vi "Read Last Known State.vi"(8 "error in (no error)":errorcluster, 11 "FP-TC-Shared.lvclass":refnum<class "FP-TC-Shared.lvclass">) -> (0 "error out":errorcluster, 1 "Last State Known":bool, 2 "LC Type":T1, 3 "FP-TC-Shared.lvclass":refnum<class "FP-TC-Shared.lvclass">)   [LabVIEW 2019, in "FP-TC-Shared.lvclass"]
uses:
  FP-TC-Shared.lvclass
  typedefs/LC Type--Enum.ctl
  FP-TC-Shared.lvclass/FP-TC-Shared.ctl
  <vilib>/Utility/config.llb/NI_LVConfig.lvlib
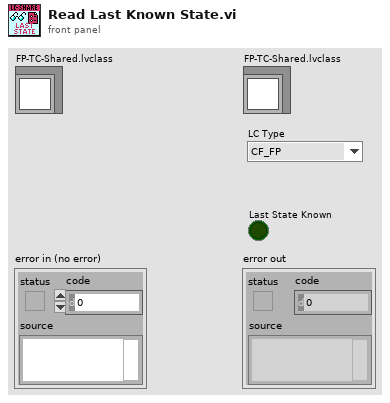
[diagram p1: front panel]
types:
  T1 = typedef "FP-TC-Shared.lvclass/LC Type--Enum.ctl" = enum16{"CF_FP", "CF_TC", "CF_TC_Z", "MNK_FP", "MNK_TC", "MNK_TC_Z", "unknown"}
  T2 = typedef "FP-TC-Shared.lvclass/Configuration--Cluster.ctl" = cluster{"Application":enum16{"TC", "FP"}, "LC Type":T1}
  T3 = typedef "NI_LVConfig.lvlib/Config Data RefNum.ctl" = refnum<k1>
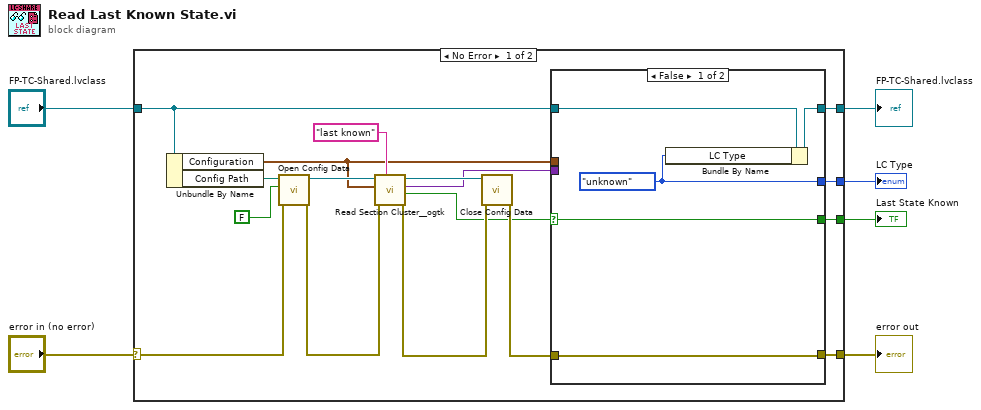
[diagram p0: block diagram]
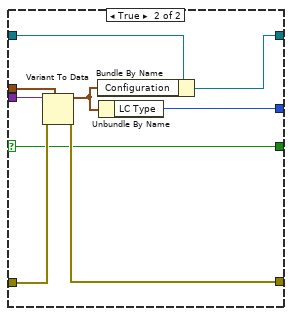
[diagram p2: hidden frame]
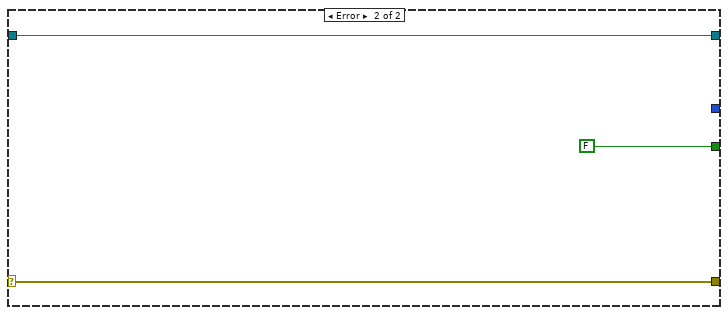
[diagram p3: hidden frame]
diagram:
  n1 = case shown="No Error" "error in (no error)" {
    selector: "error in (no error)" -> [w20 w40]
    tunnel: [w11 w40] -> w5
    tunnel: [w23 w39] -> w3
    tunnel: "FP-TC-Shared.lvclass" -> [w22 w39]
    tunnel: [w9 FALSE ("all found?")] -> w2
    tunnel: [w8 _] -> w1
    frame No Error {
      n2 = Unbundle By Name(w22) -> ("Configuration"=w15:T2, "Config Path"=w21:path)
      n3 = call <vilib>:"Open Config Data.vi"("error in (no error)"=w20, "create file if necessary (T)"=FALSE, "configuration file path"=w21) -> ("error out"=w16:errorcluster, "refnum"=w18:T3)  [unwired: 6 in, 1 out]
      n4 = call <userlib>:"Read Section Cluster__ogtk.vi"("section (optional)"="last known" ("regular expression"), "error in (no error)"=w16, "Section Formatted Cluster Type"=w15, "refnum"=w18) -> ("error out"=w13:errorcluster, "all found?"=w10:bool, "Section Formatted Cluster"=w14:variant, "dup refnum"=w17:T3)  [unwired: 3 in, 1 out]
      n5 = call <vilib>:"Close Config Data.vi"("error in (no error)"=w13, "refnum"=w17) -> ("error out"=w12:errorcluster)  [unwired: 8 in, 1 out]
      n6 = case shown="False" w10 {
        selector: w10 -> [w28 w31]
        tunnel: [w25 w37] -> w23
        tunnel: w22 -> [w24 w36]
        tunnel: w15 -> [_ w35]
        tunnel: w14 -> [_ w34]
        tunnel: w12 -> [w27 w33]
        tunnel: [w27 w32] -> w11
        tunnel: [w28 w31] -> w9
        tunnel: [w26 w29] -> w8
        frame False {
          w26 = LC_Type--Enum."unknown" ("LC Type")
          n7 = Bundle By Name(cluster=w24, "LC Type"=w26) -> (w25:refnum<class "FP-TC-Shared.lvclass">)
        }
        frame True {
          n8 = Variant To Data(error in=w33, type=w35, Variant=w34) -> (data=w30:T2, error out=w32:errorcluster)
          n9 = Bundle By Name(cluster=w36, "Configuration"=w30) -> (w37:refnum<class "FP-TC-Shared.lvclass">)
          n10 = Unbundle By Name(w30) -> ("LC Type"=w29:T1)
        }
      }
    }
    frame Error {
    }
  }
  "error out" <- w5
  "FP-TC-Shared.lvclass" <- w3
  "Last State Known" <- w2
  "LC Type" <- w1
